vi "Main.vi"() -> ()   [LabVIEW 2012]
uses:
  <vilib>/Instr/_visa.llb/VISA Configure Serial Port (Instr).vi
panel:
  out "Z2":dbl[](graph)
  out "Y2":dbl[](graph)
  out "X2":dbl[](graph)
  out "Z1":dbl[](graph)
  out "Y1":dbl[](graph)
  out "X1":dbl[](graph)
  # "PMT Channel 1"
  # "PMT Channel 2"
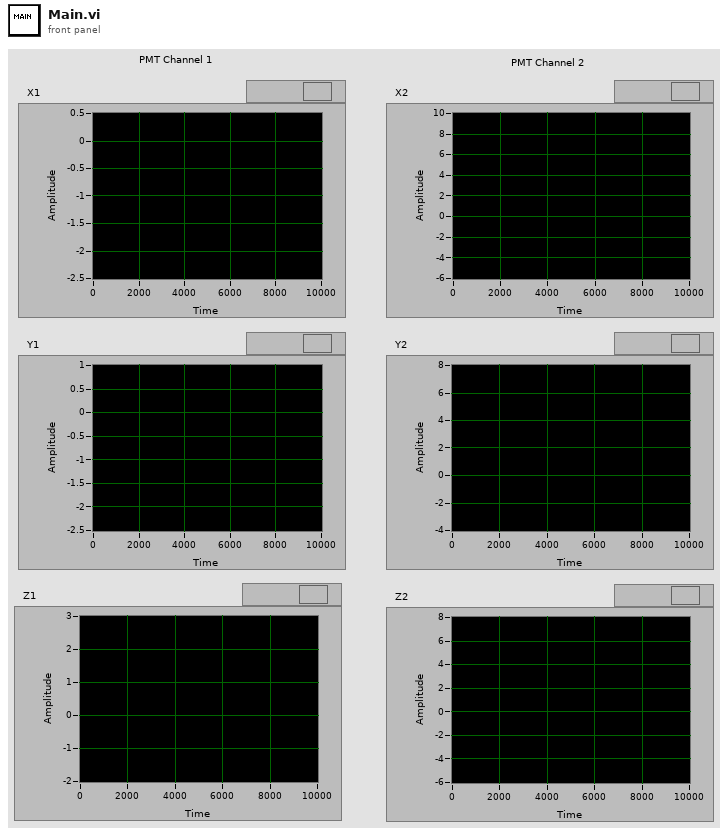
[diagram p1: front panel]
types:
  T1 = cluster{"PMTChans":i32, "NumScanPlanes":i32, "ScanRows":i32, "ScanCols":i32, "NumSamples":i32}
  T2 = cluster{"Dx_drow":dbl, "Dy_drow":dbl, "Dz_drow":dbl, "Dx_dcol":dbl, "Dy_dcol":dbl, "Dz_dcol":dbl}
  T3 = cluster{"X1":dbl[], "Y1":dbl[], "Z1":dbl[], "X2":dbl[], "Y2":dbl[], "Z2":dbl[]}
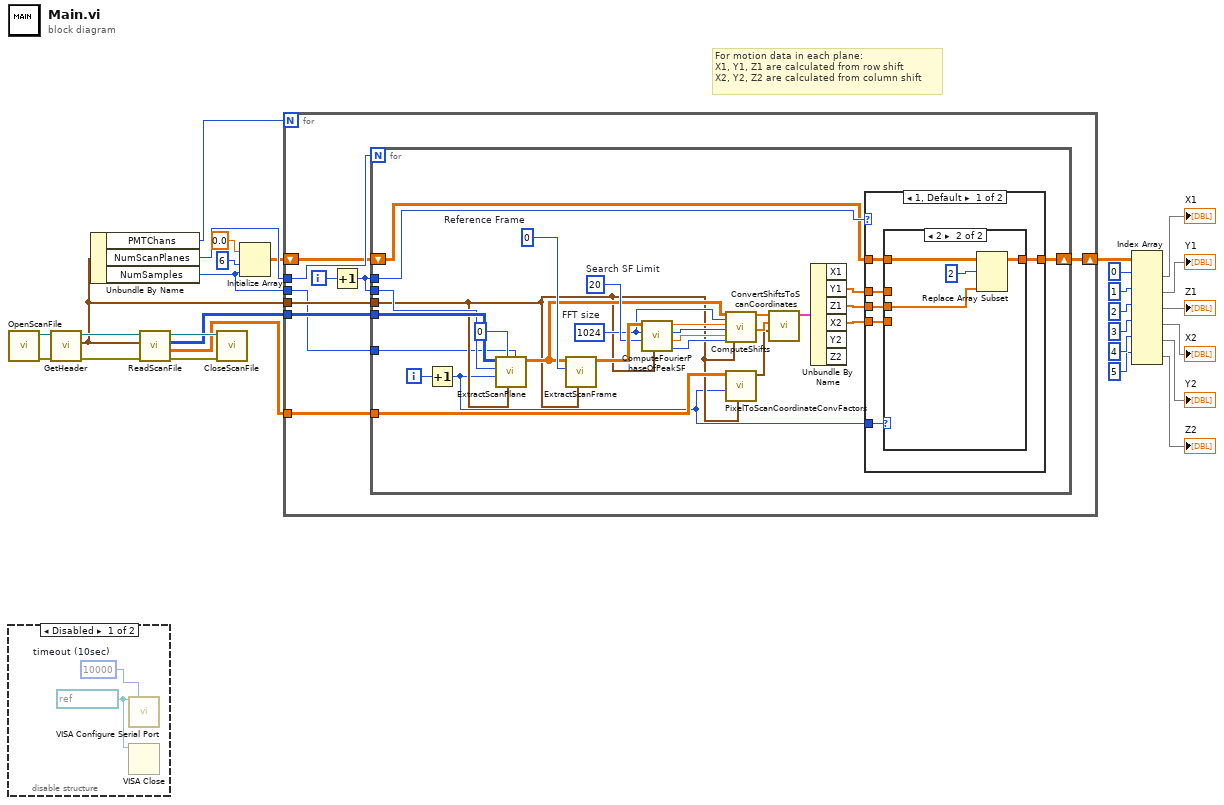
[diagram p0: block diagram]
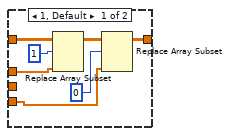
[diagram p2: hidden frame]
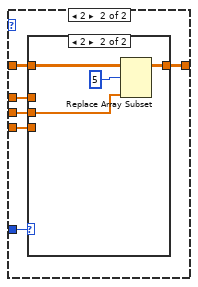
[diagram p3: hidden frame]
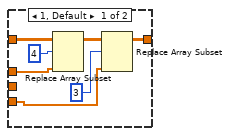
[diagram p4: hidden frame]
diagram:
  # "For motion data in each plane:\nX1, Y1, Z1 are calculated from row shift\nX2, Y2, Z2 are calculated from column shift"
  n1 = call "OpenScanFile.vi"() -> ("error out"=w27:errorcluster, "refnum out"=w28:refnum<file>)  [unwired: 10 in]
  n2 = disable-structure shown="Disabled" {
    frame Disabled {
      w29 = refnum<visa-resource-name> "COM1" ("VISA resource name")
      w30 = u32 10000  # timeout (10sec)
      n3 = call-poly "VISA Configure Serial Port"("VISA resource name"=w29, "timeout (10sec)"=w30) -> ()  [unwired: 7 in, 7 out]
      n4 = VISA Close(VISA resource name=w29) -> ()  [unwired: 1 in, 1 out]
    }
    frame Enabled {
    }
  }
  n5 = call "GetHeader.vi"("error in"=w27, "refnum in"=w28) -> ("error out"=w23:errorcluster, "Header"=w20:T1, "refnum out"=w26:refnum<file>)  [unwired: 6 in]
  n6 = Unbundle By Name(w20) -> ("PMTChans"=w18:i32, "NumScanPlanes"=w19:i32, "NumSamples"=w1:i32)
  n7 = call "ReadScanFile.vi"("error in"=w23, "Header"=w20, "refnum in"=w26) -> ("error out"=w24:errorcluster, "Coordinate Data"=w21:dbl[][][][], "Scan Data"=w22:i32[][][][], "refnum out"=w25:refnum<file>)  [unwired: 5 in]
  n8 = call "CloseScanFile.vi"("error in"=w24, "refnum"=w25) -> ()  [unwired: 9 in, 1 out]
  n9 = Initialize Array(0.0 ("element"), 6 ("dimension size"), w1) -> (w16:dbl[][])
  n10 = for {
    N: w18 -> [_]
    tunnel: w22 -> [w39]
    tunnel: w21 -> [w38]
    tunnel: w20 -> [w37]
    tunnel: w19 -> [w36]
    shift-right: [w32] -> w2
    shift-left: w16 -> [w33]
    tunnel: w1 -> [w31]
    i -> [w35]
    n11 = Increment(x=w35) -> (x+1=w34:i32)
    n12 = for {
      N: w36 -> [_]
      tunnel: w39 -> [w66]
      tunnel: w34 -> [w65]
      tunnel: w38 -> [w55]
      tunnel: w37 -> [w54]
      tunnel: w34 -> [w47]
      shift-right: [w42] -> w32
      shift-left: w33 -> [w46]
      tunnel: w31 -> [w40]
      i -> [w49]
      w62 = 20  # Search SF Limit
      w60 = 1024  # FFT size
      w64 = 0  # Reference Frame
      n13 = Increment(x=w49) -> (x+1=w48:i32)
      n14 = call "ExtractScanPlane.vi"("End Frame"=w40, "Header"=w54, "Start Frame"=0, "Scan Plane"=w48, "PMT Channel"=w65, "All Scan Data"=w66) -> ("Scan Plane Data"=w61:dbl[][][])  [unwired: 5 in]
      n15 = call "ExtractScanFrame.vi"("Header"=w54, "Scan Frame"=w64, "Scan Plane Data"=w61) -> ("Scan Frame Data"=w63:dbl[][])  [unwired: 8 in]
      n16 = call "ComputeFourierPhaseOfPeakSF.vi"("Header"=w54, "Search SF Limit"=w62, "FFT size"=w60, "Scan Frame"=w63) -> ("Col Shift Element Number"=w56:i32, "Vertical SF Phase"=w57:dbl, "Row Shift Element Numbert"=w58:i32, "Horizontal SF Phase"=w59:dbl)  [unwired: 4 in]
      n17 = call "ComputeShifts.vi"("Scan Plane Data"=w61, "FFT size"=w60, "Ref Horizontal SF Phase"=w59, "Ref Row Shift Element"=w58, "Ref Vertical SF Phase"=w57, "Ref Col Shift Element"=w56, "Header"=w54) -> ("Row Shift Array"=w53:dbl[], "Col Shift Array"=w52:dbl[])  [unwired: 11 in]
      n18 = call "PixelToScanCoordinateConvFactors.vi"("Header"=w54, "Scan Plane"=w48, "Coordinate Data"=w55) -> ("PixelToScanCoordConvFactors"=w51:T2)  [unwired: 8 in]
      n19 = call "ConvertShiftsToScanCoordinates.vi"("PixelToScanCoordConvFactors"=w51, "Col Shift Array"=w52, "Row Shift Array"=w53) -> ("Motion"=w50:T3)  [unwired: 8 in]
      n20 = Unbundle By Name(w50) -> ("Y1"=w44:dbl[], "Z1"=w43:dbl[], "X2"=w45:dbl[])  [unwired: 3 out]
      n21 = case shown="1, Default" w47 {
        tunnel: w48 -> [w72 w89]
        tunnel: w46 -> [w71 w88]
        tunnel: w45 -> [w70 w87]
        tunnel: w44 -> [w69 w86]
        tunnel: w43 -> [w68 w85]
        tunnel: [w67 w84] -> w42
        frame 1, Default {
          n22 = case shown="2" w72 {
            tunnel: w71 -> [w79 w83]
            tunnel: w70 -> [w77 _]
            tunnel: w69 -> [w75 _]
            tunnel: w68 -> [_ w81]
            tunnel: [w73 w80] -> w67
            frame 1, Default {
              n23 = Replace Array Subset(array=w79, new element=w75, index (row)=1) -> (w74:dbl[][])  [unwired: 1 in]
              n24 = Replace Array Subset(array=w74, new element=w77, index (row)=0) -> (w73:dbl[][])  [unwired: 1 in]
            }
            frame 2 {
              n25 = Replace Array Subset(array=w83, new element=w81, index (row)=2) -> (w80:dbl[][])  [unwired: 1 in]
            }
          }
        }
        frame 2 {
          n26 = case shown="2" w89 {
            tunnel: w88 -> [w94 w98]
            tunnel: w87 -> [w93 _]
            tunnel: w86 -> [w92 _]
            tunnel: w85 -> [_ w99]
            tunnel: [w90 w97] -> w84
            frame 1, Default {
              n27 = Replace Array Subset(array=w94, new element=w92, index (row)=4) -> (w91:dbl[][])  [unwired: 1 in]
              n28 = Replace Array Subset(array=w91, new element=w93, index (row)=3) -> (w90:dbl[][])  [unwired: 1 in]
            }
            frame 2 {
              n29 = Replace Array Subset(array=w98, new element=w99, index (row)=5) -> (w97:dbl[][])  [unwired: 1 in]
            }
          }
        }
      }
    }
  }
  n30 = Index Array(array=w2, index (row) #1=0 ("index (row)"), index (row) #2=1 ("index (row)"), index (row) #3=2 ("index (row)"), index (row) #4=3 ("index (row)"), index (row) #5=4 ("index (row)"), index (row) #6=5 ("disabled index (col)")) -> (element #1=→"X1":dbl[], element #2=→"Y1":dbl[], element #3=→"Z1":dbl[], element #4=→"X2":dbl[], element #5=→"Y2":dbl[], element #6=→"Z2":dbl[])  [unwired: 6 in]
